vi "Read.vi"(7 "SFTP Attributes In":refnum<class "SFTP Attributes.lvclass">, 8 "Error In":errorcluster, 10 "Max Data Length":i32=512, 11 "SFTP Directory In":refnum<class "SFTP Directory.lvclass">) -> (0 "Error Out":errorcluster, 1 "End-of-Directory?":bool, 2 "File Name":string, 3 "SFTP Directory Out":refnum<class "SFTP Directory.lvclass">, 5 "SFTP Attributes Out":refnum<class "SFTP Attributes.lvclass">)   [LabVIEW 2018, in "Toolkit.lvlib" / "SFTP Directory.lvclass"]
uses:
  SFTP Directory.lvclass
  SFTP Attributes/SFTP Attributes.lvclass
  SFTP Directory.lvclass/SFTP Directory.ctl
  SFTP Attributes/SFTP Attributes.lvclass/SFTP Attributes.ctl
  SFTP/SFTP.lvclass/SFTP.ctl
  Session/Session.lvclass/Session.ctl
  SSH/SSH.lvclass/SSH.ctl
  Toolkit.lvlib
  SFTP/SFTP.lvclass
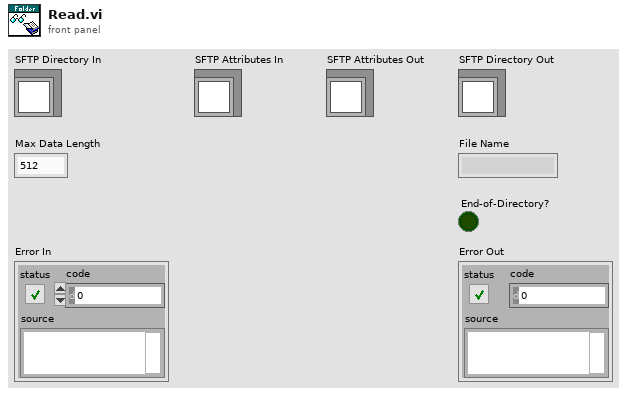
[diagram p1: front panel]
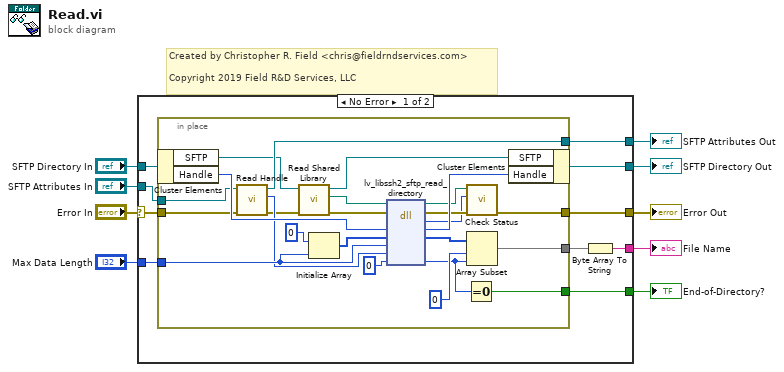
[diagram p0: block diagram]
diagram:
  # "Created by Christopher R. Field <chris@fieldrndservices.com>\n\nCopyright 2019 Field R&D Services, LLC"
  n1 = case shown="No Error" "Error In" {
    selector: "Error In" -> [w18 w45]
    tunnel: "SFTP Directory In" -> [w19 w46]
    tunnel: [w17 w46] -> w5
    tunnel: [w16 w45] -> w8
    tunnel: "Max Data Length" -> [w15 _]
    tunnel: "SFTP Attributes In" -> [w14 w44]
    tunnel: [w13 w44] -> w3
    tunnel: [w12 _] -> w2
    tunnel: [w10 _] -> w1
    frame No Error {
      n2 = in-place {
        in-place-border: w18 -> [w31]
        in-place-border: [w39] -> w16
        in-place-border: [w32] -> w11
        in-place-border: w15 -> [w36]
        in-place-border: w14 -> [w30]
        in-place-border: [w27] -> w13
        in-place-border: [w24] -> w12
        n3 = in-place-cluster #1(w19) -> ("SFTP"=w22:refnum<class "SFTP.lvclass">, "Handle"=w43:u64)
        n4 = call "Read Handle.vi"("Error In"=w31, "SFTP Attributes In"=w30) -> ("Error Out"=w28:errorcluster, "Handle"=w29:u64, "SFTP Attributes Out"=w27:refnum<class "SFTP Attributes.lvclass">)  [unwired: 7 in]
        n5 = call "Read Shared Library.vi"("Error In"=w28, "SFTP In"=w22) -> ("Erorr Out"=w23:errorcluster, "libssh2lv Shared Library"=w20:path, "SFTP Out"=w21:refnum<class "SFTP.lvclass">)  [unwired: 7 in]
        n6 = Initialize Array(u8 0, w36) -> (w37:u8[])
        n7 = dll-call lib="lv-libssh2.*" fn="lv_libssh2_sftp_read_directory"(path in=w20, error in=w23, "handle"=w43, "buffer"=w37, "buffer_max_length"=w36, "attributes"=w29, "read_count"=i64 0) -> (path out=w40:path, error out=w41:errorcluster, "status"=w26:i32, "handle"=w42:u64, "buffer"=w34:u8[], "read_count"=w25:i64)  [unwired: 3 in]
        n8 = Equal To 0?(x=w25) -> (x = 0?=w24:bool)
        n9 = call "Check Status.vi"("Error In"=w41, "Status"=w26, "lv-libssh2 Shared Library In"=w40) -> ("Error Out"=w39:errorcluster)  [unwired: 7 in, 1 out]
        n10 = Array Subset(array=w34, index=0, length=w25) -> (w32:u8[])
        n11 = in-place-cluster #1("SFTP"=w21, "Handle"=w42) -> (w17:refnum<class "SFTP Directory.lvclass">)
      }
      n12 = Byte Array To String(unsigned byte array=w11) -> (string=w10:string)
    }
    frame Error {
    }
  }
  "Error Out" <- w8
  "End-of-Directory?" <- w2
  "SFTP Directory Out" <- w5
  "SFTP Attributes Out" <- w3
  "File Name" <- w1
